vi "CH0_Manual_range_select.vi"(9 "Select COM port":refnum<visa-resource-name>="COM3", 10 "EN":bool, 11 "IN1 L":u8(knob) scale=0.0..3.0) -> (3 "CH0 IN1 L":string)   [LabVIEW 2012]
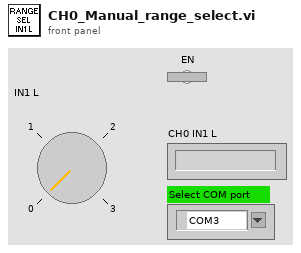
[diagram p1: front panel]
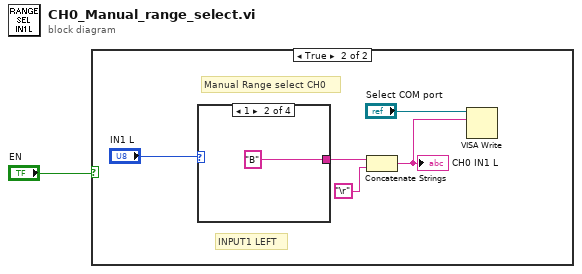
[diagram p0: block diagram]
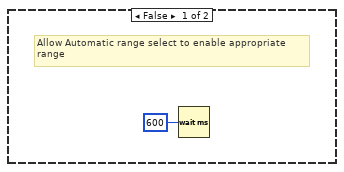
[diagram p2: hidden frame]
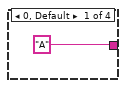
[diagram p3: hidden frame]
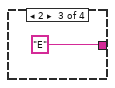
[diagram p4: hidden frame]
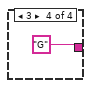
[diagram p5: hidden frame]
diagram:
  n1 = case shown="True" "EN" {
    frame False {
      # "Allow Automatic range select to enable appropriate\nrange"
      n2 = Wait (ms)(milliseconds to wait=600) -> ()  [unwired: 1 out]
    }
    frame True {
      # "INPUT1 LEFT"
      # "Manual Range select CH0"
      n3 = case shown="1" "IN1 L" {
        tunnel: ["A" "B" "E" "G"] -> w6
        frame 0, Default {
        }
        frame 1 {
        }
        frame 2 {
        }
        frame 3 {
        }
      }
      n4 = Concatenate Strings(w6, "\r") -> (w3:string)
      "CH0 IN1 L" <- w3
      n5 = VISA Write(VISA resource name="Select COM port", write buffer=w3) -> ()  [unwired: 1 in, 3 out]
    }
  }
